vi "RSZVB Marker Bandfilter Results.vi"(0 "VISA session":refnum<visa-resource-name>, 5 "Channel (Trace) (1)":i32=1, 7 "Marker (1)":i32=1, 11 "error in (no error)":errorcluster {"code" format="%.0x"}) -> (2 "UBE":dbl format="%^.3e", 3 "Loss":dbl format="%^.3e", 4 "dup VISA session":refnum<visa-resource-name>, 6 "Q":dbl format="%^.3e", 8 "Bandwidth":dbl format="%^.3e", 10 "Center Stimulus":dbl format="%^.3e", 14 "LBE":dbl format="%^.3e", 15 "error out":errorcluster {"code" format="%.0x"})   [LabVIEW 2011]
doc: "This VI returns the results of a bandpass or a bandstop filter search. Result is only available after a bandfilter search has been executed.\n\nNote(s):\n\nUnits of the result values depends on the sweep type and the marker format; see CALCulate<Ch/Tr>:MARKer<Mk>:FORMat.\n\nRemote-control command(s):\nCALCulate<Ch/Tr>:MARKer<Mk>:BWIDth?"
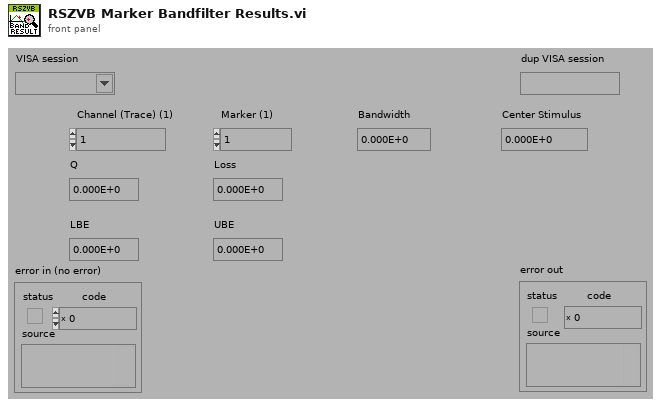
[diagram p1: front panel]
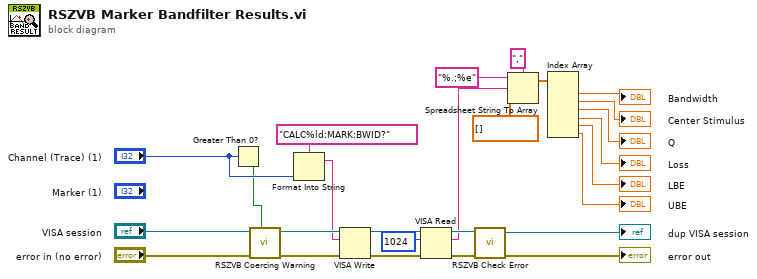
[diagram p0: block diagram]
diagram:
  n1 = Greater Than 0?(x="Channel (Trace) (1)") -> (x > 0?=w1:bool)
  n2 = call "RSZVB Coercing Warning.vi"("In Range?"=w1, "error in (no error)"="error in (no error)", "VISA session"="VISA session") -> ("error out"=w21:errorcluster, "dup VISA session"=w22:refnum<visa-resource-name>)  [unwired: 7 in]
  n3 = Format Into String(format string="CALC%ld:MARK:BWID?", "Channel (Trace) (1)") -> (resulting string=w20:string)  [unwired: 2 in, 1 out]
  n4 = VISA Write(VISA resource name=w22, write buffer=w20, error in (no error)=w21) -> (VISA resource name out=w18:refnum<visa-resource-name>, error out=w19:errorcluster)  [unwired: 1 out]
  n5 = VISA Read(VISA resource name=w18, byte count=u32 1024 ("byte count (0)"), error in (no error)=w19) -> (VISA resource name out=w25:refnum<visa-resource-name>, read buffer=w12:string, error out=w24:errorcluster)  [unwired: 1 out]
  n6 = call "RSZVB Check Error.vi"("error in (no error)"=w24, "VISA session"=w25) -> ("error out"=→"error out":errorcluster, "dup VISA session"=→"dup VISA session":refnum<visa-resource-name>)  [unwired: 8 in]
  n7 = Spreadsheet String To Array(delimiter (Tab)=",", format string="%.;%e", spreadsheet string=w12, array type (2D Dbl)=dbl[] []) -> (array=w8:dbl[])
  n8 = Index Array(array=w8) -> (element #1=→"Bandwidth":dbl, element #2=→"Center Stimulus":dbl, element #3=→"Q":dbl, element #4=→"Loss":dbl, element #5=→"LBE":dbl, element #6=→"UBE":dbl)  [unwired: 6 in]
